vi "SiosIfmSetHumidity.vi"(0 "Humidity":dbl, 1 "Channel":i32(knob) scale=1.0..4.0, 2 "Device Number":i32) -> ()   [LabVIEW 2009]
uses:
  siosifm.dll
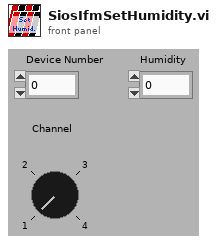
[diagram p1: front panel]
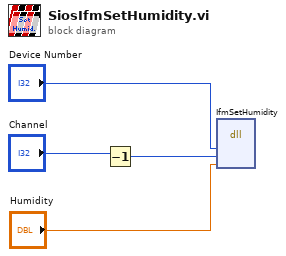
[diagram p0: block diagram]
diagram:
  n1 = Decrement(x="Channel") -> (x-1=w3:i32)
  n2 = dll-call lib="C:/WORK/Artem/RE-10/SIOS_IfmDLL/siosifm.dll" fn="IfmSetHumidity"("devNumber"="Device Number", "Channel"=w3, "Humidity"="Humidity") -> ()  [unwired: 7 in, 2 out]
